vi "Sam_OpenVINO.vi"() -> ()   [LabVIEW 2018]
doc: "Sam_OpenVINO: This example is an example of using the SAM model to achieve semantic segmentation. The SAM model is a semantic segmentation model based on Convolutional Neural Networks (CNN). It adopts technologies such as multi-scale feature fusion and context information encoding, which can achieve pixel level fine segmentation. In this example, by loading the image and clicking on the segmentation area, the segmentation of the region of interest can be achieved."
uses:
  vi.lib/VIRobotics/opencv_yiku/ctls/ColorConversionCodes.ctl
  vi.lib/VIRobotics/opencv_yiku/Mat/Mat_8U/Mat_8U.lvclass
  C:/Program Files/National Instruments/LabVIEW 2018/vi.lib/VIRobotics/opencv_yiku/Mat/Mat/Mat.lvclass
  vi.lib/VIRobotics/ModelZoo/Segmentation/Segment_Anything_OpenVINO/Segment_Anything_OpenVINO.lvclass
  C:/Program Files/National Instruments/LabVIEW 2018/vi.lib/VIRobotics/ModelZoo/Segmentation/Segment_Anything_Utils/Segment_Anything_Utils.lvclass
  vi.lib/VIRobotics/ModelZoo/Segmentation/Segment_Anything_OpenVINO/InitialModel_Segment_Anything_OpenVINO.vi
  vi.lib/VIRobotics/opencv_yiku/Mat/Create_Mat_8U.vi
  vi.lib/VIRobotics/ModelZoo/Segmentation/Segment_Anything_Utils/set_point_coords.vi
  vi.lib/VIRobotics/opencv_yiku/Mat/Create_Mat_8UC3_Size.vi
  vi.lib/VIRobotics/opencv_yiku/Mat/Mat/Mat_release.vi
  vi.lib/VIRobotics/opencv_yiku/Mat/Mat/Mat.lvclass
  vi.lib/VIRobotics/opencv_yiku/opencv_yiku.lvlib
  vi.lib/VIRobotics/ModelZoo/Segmentation/Segment_Anything_Utils/Segment_Anything_Utils.lvclass
panel:
  in  "decodr_config":cluster{"decoder_model":path, "device":string}={"decoder_model"=path "C:/ProgramData/VIRobotics/ModelZoo/Segmentation/sam/sam-b-dec.onnx", "device"="CPU"}
  in  "encoder_config":cluster{"encoder_model":path, "device":string}={"encoder_model"=path "C:/ProgramData/VIRobotics/ModelZoo/Segmentation/sam/sam-b-enc.onnx", "device"="CPU"}
  in  "img":path=path "C:/ProgramData/VIRobotics/ModelZoo/Segmentation/imgs/plant.jpg"
  out "picture":picture
  out "x-y":dbl
  out "mask":picture
  in  "run":bool
  # "Overview: Demonstrates how to use OpenVINO to load the ONNX model of sam for Semantic segmentation annotation\nRequirements: Windows.\nInstructions: \n1.Run the VI.\n2.Specify the img that requires segmentation annotation。\n3.Click on the target with the mouse on the picture control\n4.Click run"
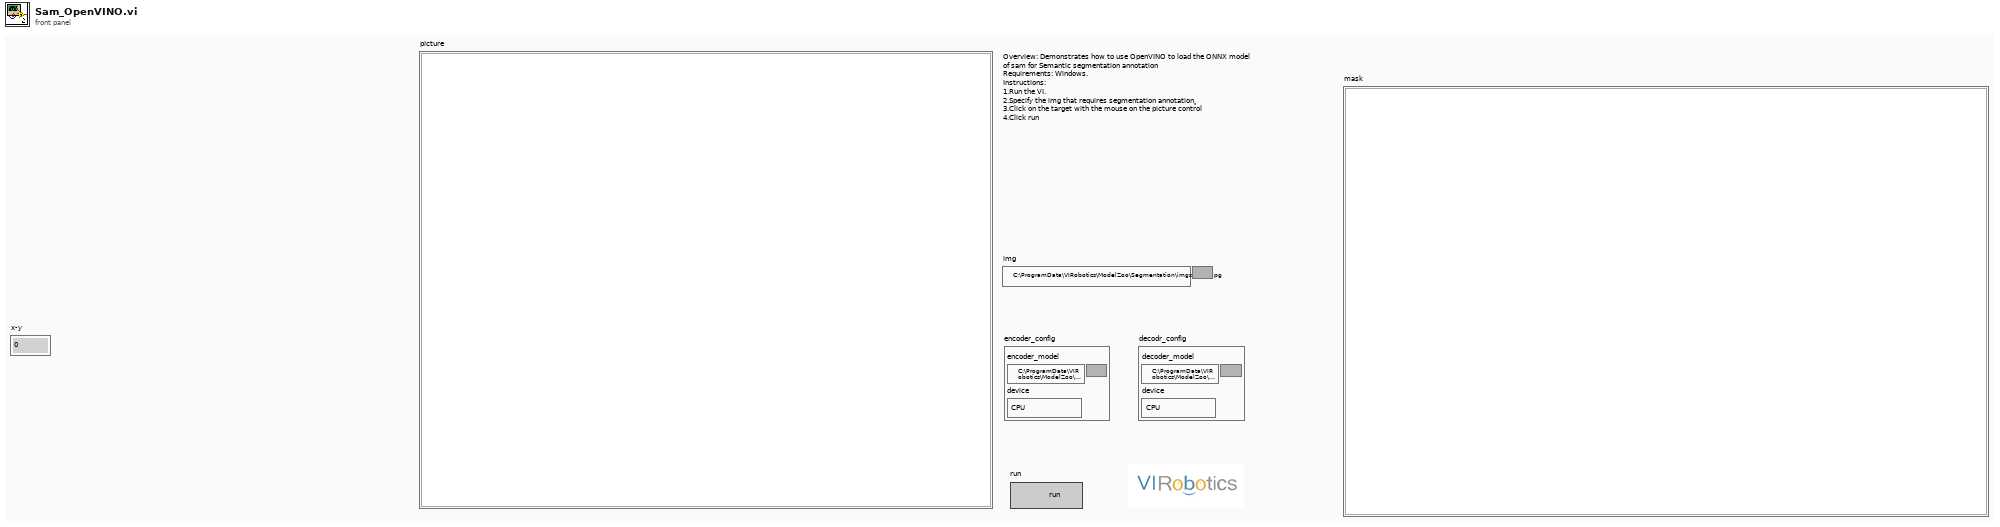
[diagram p1: front panel]
types:
  T1 = typedef "opencv_yiku.lvlib/ColorConversionCodes.ctl" = enum32{"COLOR_BGR2BGRA", "COLOR_BGRA2BGR", "COLOR_BGR2RGBA", "COLOR_RGBA2BGR", "COLOR_BGR2RGB", "COLOR_BGRA2RGBA", "COLOR_BGR2GRAY", "COLOR_RGB2GRAY", "COLOR_GRAY2BGR", "COLOR_GRAY2BGRA", "COLOR_BGRA2GRAY", "COLOR_RGBA2GRAY", "COLOR_BGR2BGR565", "COLOR_RGB2BGR565", "COLOR_BGR5652BGR", "COLOR_BGR5652RGB", "COLOR_BGRA2BGR565", "COLOR_RGBA2BGR565", "COLOR_BGR5652BGRA", "COLOR_BGR5652RGBA", "COLOR_GRAY2BGR565", "COLOR_BGR5652GRAY", "COLOR_BGR2BGR555", "COLOR_RGB2BGR555", "COLOR_BGR5552BGR", "COLOR_BGR5552RGB", "COLOR_BGRA2BGR555", "COLOR_RGBA2BGR555", "COLOR_BGR5552BGRA", "COLOR_BGR5552RGBA", "COLOR_GRAY2BGR555", "COLOR_BGR5552GRAY", "COLOR_BGR2XYZ", "COLOR_RGB2XYZ", "COLOR_XYZ2BGR", "COLOR_XYZ2RGB", "COLOR_BGR2YCrCb", "COLOR_RGB2YCrCb", "COLOR_YCrCb2BGR", "COLOR_YCrCb2RGB", "COLOR_BGR2HSV", "COLOR_RGB2HSV", "42", "43", "COLOR_BGR2Lab", "COLOR_RGB2Lab"}
  T2 = typedef "LVBoundsTypeDef.ctl" = cluster{"Width":u32, "Height":u32}
  T3 = typedef "LVMouseTypeDef.ctl" = cluster{"Mouse Position":cluster{"X":i32, "Y":i32}, "Mouse Modifiers":cluster{"Button Down":bool, "Shift Mod":bool, "Menu Mod":bool, "Option Mod":bool}}
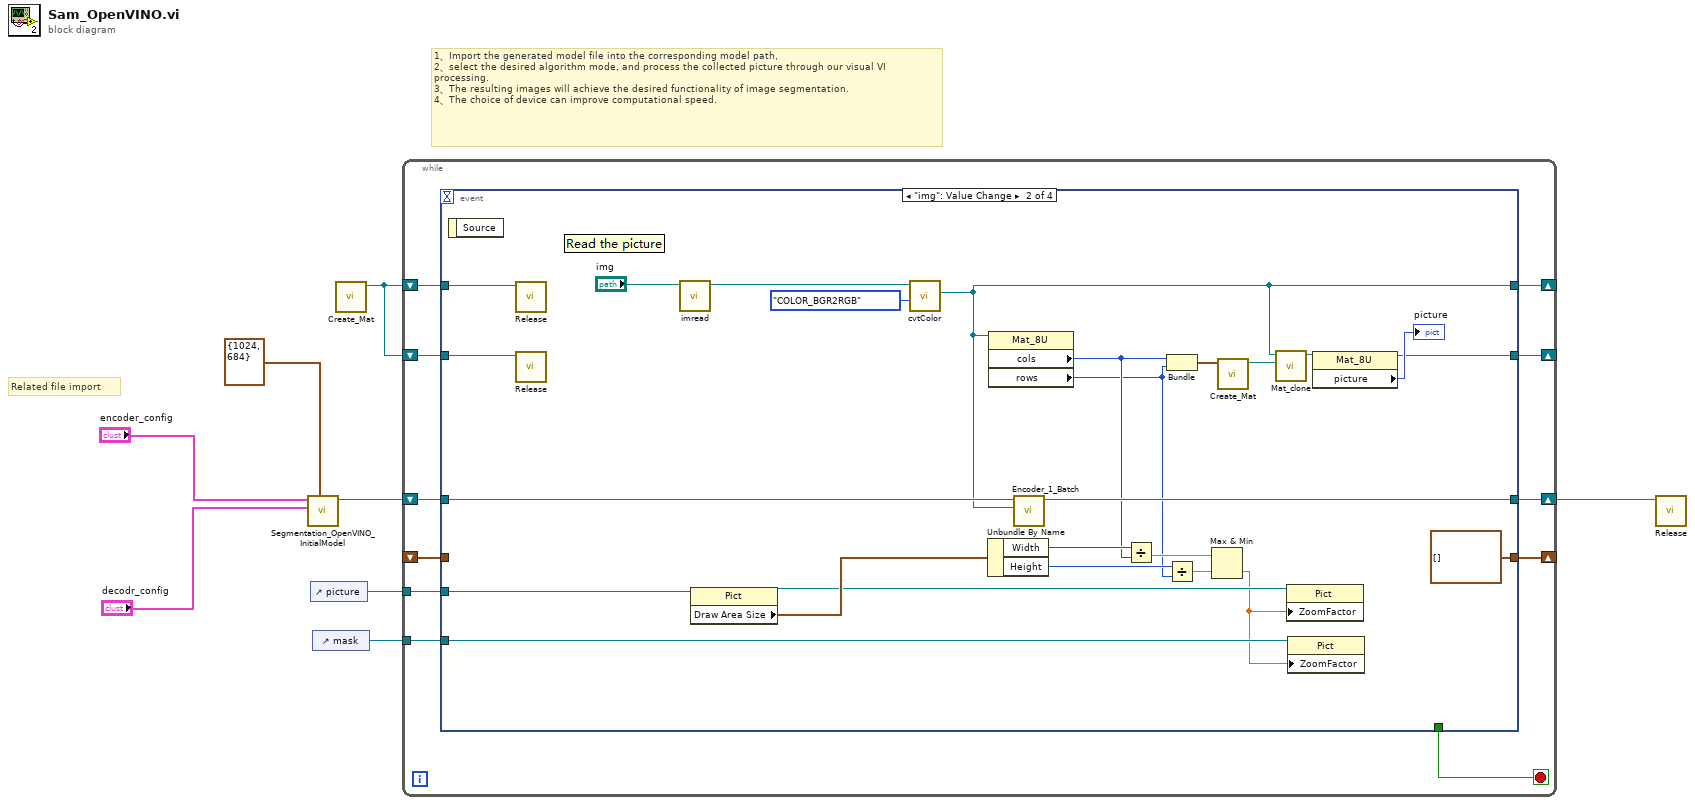
[diagram p0: block diagram]
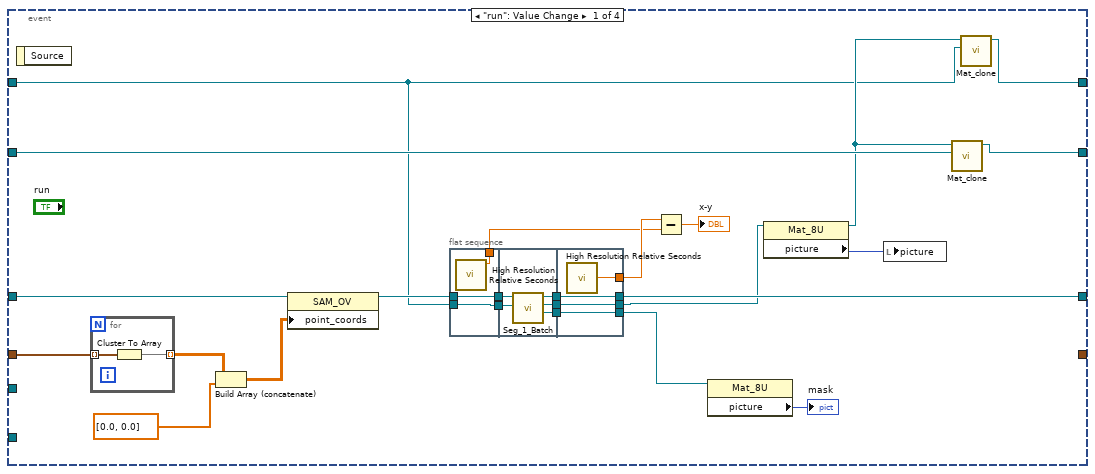
[diagram p2: hidden frame]
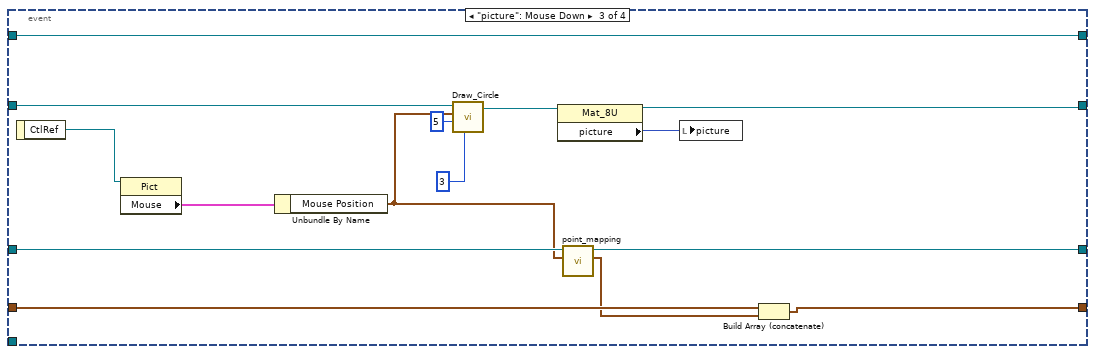
[diagram p3: hidden frame]
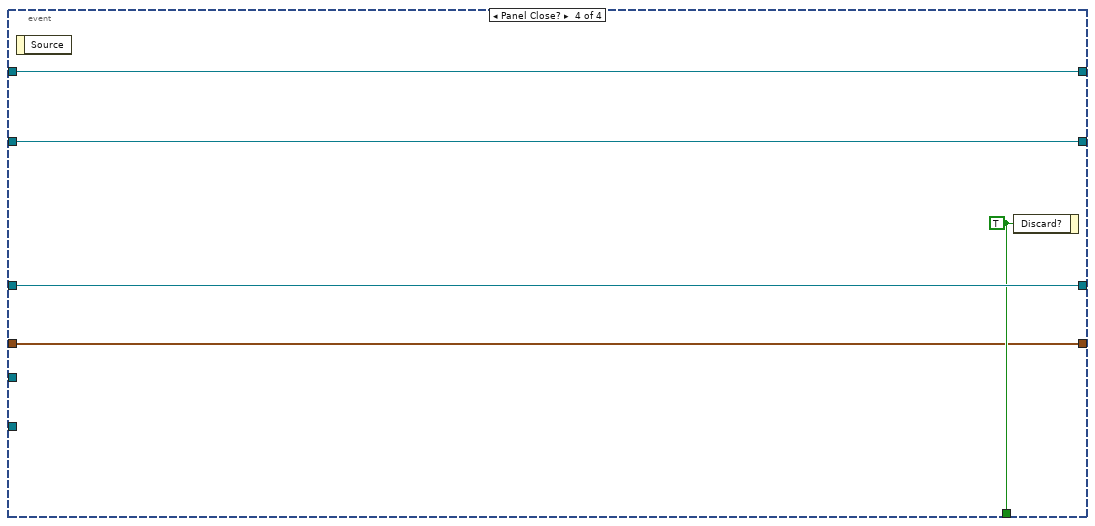
[diagram p4: hidden frame]
diagram:
  # "1、Import the generated model file into the corresponding model path, \n2、select the desired algorithm mode, and process the collected picture through our visual VI processing. \n3、The resulting images will achieve the desired functionality of image segmentation. \n4、The choice of device can improve computational speed."
  # "Related file import"
  n1 = call-poly "Segmentation_OpenVINO_InitialModel.vi"("inputSize"=cluster{"x":i32, "y":i32} {"x"=1024, "y"=684} ("Size"), "decodr_config"="decodr_config", "encoder_config"="encoder_config") -> ("SAM_OV out"=w4:refnum<class "Segment_Anything_OpenVINO.lvclass">)  [unwired: 7 in, 1 out]
  n2 = control-ref of="picture"() -> (w7:refnum<vi>)
  n3 = control-ref of="mask"() -> (w6:refnum<vi>)
  n4 = call-poly "Create_Mat.vi"() -> ("Mat_8U_out"=w5:refnum<class "Mat_8U.lvclass">)  [unwired: 10 in, 1 out]
  n5 = while {
    shift-right: [w18] -> w8
    shift-left: w4 -> [w19]
    tunnel: w7 -> [w16]
    shift-right: [w15] -> _
    shift-left: w5 -> [w14]
    tunnel: w6 -> [w13]
    shift-right: [w12] -> _
    shift-left: _ -> [w11]
    shift-right: [w10] -> _
    shift-left: w5 -> [w9]
    stop <- w17 stop-if-true
    n6 = event shown="[1] \"img\": Value Change" {
      selector: _ -> [_ _ _ _]
      dyn-events: _ -> [_ _ _ _]
      timeout: _ -> [_ _ _ _]
      tunnel: w19 -> [w34 w81 w86 w102]
      tunnel: [w32 w80 w85 w102] -> w18
      tunnel: [_ _ _ w101] -> w17
      tunnel: w16 -> [_ w77 _ _]
      tunnel: [w21 w64 w96 w99] -> w15
      tunnel: w14 -> [w22 w70 w96 w99]
      tunnel: w13 -> [_ w59 _ _]
      tunnel: [_ cluster{"x":sgl, "y":sgl}[] [] w89 w100] -> w12
      tunnel: w11 -> [w31 _ w90 w100]
      tunnel: [w24 w61 w87 w98] -> w10
      tunnel: w9 -> [w25 w60 w88 w98]
      event "run": Value Change {
        n7 = event-data() -> ()  [unwired: 1 in, 1 out]
        n8 = for {
          tunnel: w31 -> [w45] mode=indexing
          tunnel: [w44] -> w30 mode=indexing
          n9 = Cluster To Array(cluster=w45) -> (array=w44:sgl[])
        }
        n10 = Build Array (concatenate)(w30, sgl[] [0.0, 0.0] ("array")) -> (w20:sgl[][])
        n11 = property class="SAM_OV"(reference=w34, "point_coords"=w20) -> (reference out=w33:refnum<class "Segment_Anything_OpenVINO.lvclass">)  [unwired: 1 in, 1 out]
        n12 = flat-sequence {
          tunnel: w33 -> [w48]
          tunnel: [w48] -> w43
          tunnel: [w47] -> w38
          tunnel: w22 -> [w46]
          tunnel: [w46] -> w28
          tunnel: w43 -> [w53]
          tunnel: [w52] -> w42
          tunnel: [w51] -> w41
          tunnel: [w50] -> w40
          tunnel: w28 -> [w49]
          tunnel: [w56] -> w27
          tunnel: [w57] -> w32
          tunnel: w42 -> [w57]
          tunnel: w41 -> [w56]
          tunnel: [w55] -> w39
          tunnel: [w54] -> w36
          tunnel: w40 -> [w54]
          frame #0 {
            n13 = call <vilib>:"High Resolution Relative Seconds.vi"() -> ("relative seconds"=w47:dbl)
          }
          frame #1 {
            n14 = call-dynamic "Seg_1_Batch.vi"("img"=w49, "Segment_Anything_OpenVINO in"=w53) -> ("mask"=w50:refnum<class "Mat_8U.lvclass">, "img out"=w51:refnum<class "Mat_8U.lvclass">, "Segment_Anything_OpenVINO out"=w52:refnum<class "Segment_Anything_OpenVINO.lvclass">)  [unwired: 6 in, 1 out]
          }
          frame #2 {
            n15 = call <vilib>:"High Resolution Relative Seconds.vi"() -> ("relative seconds"=w55:dbl)
          }
        }
        n16 = Subtract(x=w39, y=w38) -> (x-y=→"x-y":dbl)
        n17 = property class="Mat_8U"(reference=w36) -> ("picture"=→"mask":picture)  [unwired: 1 in, 2 out]
        n18 = property class="Mat_8U"(reference=w27) -> (reference out=w23:refnum<class "Mat_8U.lvclass">, "picture"=w26:picture)  [unwired: 1 in, 1 out]
        n19 = local write "picture"(w26) -> ()
        n20 = call "Mat_clone.vi"("dst"=w25, "Mat in"=w23) -> ("dst 2"=w24:refnum<class "Mat_8U.lvclass">)  [unwired: 8 in, 1 out]
        n21 = call "Mat_clone.vi"("dst"=w22, "Mat in"=w23) -> ("dst 2"=w21:refnum<class "Mat_8U.lvclass">)  [unwired: 8 in, 1 out]
      }
      event "img": Value Change {
        n22 = event-data() -> ()  [unwired: 1 in, 1 out]
        n23 = call-poly "Release.vi"("Mat in"=w70) -> ()  [unwired: 10 in, 1 out]
        n24 = call-poly "Release.vi"("Mat in"=w60) -> ()  [unwired: 10 in, 1 out]
        n25 = call "imread.vi"("path"="img") -> ("Mat out"=w79:refnum<class "Mat_8U.lvclass">)  [unwired: 9 in, 1 out]
        n26 = property class="Pict"(reference=w77) -> (reference out=w71:refnum<vi>, "Draw Area Size"=w76:T2)  [unwired: 1 in, 1 out]
        n27 = call "cvtColor.vi"("dstCn"=ColorConversionCodes."COLOR_BGR2RGB", "src"=w79) -> ("dst out"=w64:refnum<class "Mat_8U.lvclass">)  [unwired: 7 in, 2 out]
        n28 = Unbundle By Name(w76) -> ("Width"=w75:u32, "Height"=w74:u32)
        n29 = property class="Mat_8U"(reference=w64) -> ("cols"=w68:i32, "rows"=w67:i32)  [unwired: 1 in, 2 out]
        n30 = call-dynamic "Encoder_1_Batch.vi"("image"=w64, "SAM_OV in"=w81) -> ("SAM_OV out"=w80:refnum<class "Segment_Anything_OpenVINO.lvclass">)  [unwired: 8 in, 1 out]
        n31 = Divide(x=w75, y=w68) -> (x/y=w72:dbl)
        n32 = Bundle("cols"=w68, "rows"=w67) -> (w66:cluster{"cols":i32, "rows":i32})  [unwired: 1 in]
        n33 = Divide(x=w74, y=w67) -> (x/y=w73:dbl)
        n34 = Max & Min(x=w72, y=w73) -> (min(x,y)=w58:dbl)  [unwired: 1 out]
        n35 = call-poly "Create_Mat.vi"("Size"=w66) -> ("Mat_8U_out"=w65:refnum<class "Mat_8U.lvclass">)  [unwired: 9 in, 1 out]
        n36 = call "Mat_clone.vi"("dst"=w65, "Mat in"=w64) -> ("dst 2"=w63:refnum<class "Mat_8U.lvclass">)  [unwired: 8 in, 1 out]
        n37 = property class="Pict"(reference=w71, "ZoomFactor"=w58) -> ()  [unwired: 1 in, 2 out]
        n38 = property class="Pict"(reference=w59, "ZoomFactor"=w58) -> ()  [unwired: 1 in, 2 out]
        n39 = property class="Mat_8U"(reference=w63) -> (reference out=w61:refnum<class "Mat_8U.lvclass">, "picture"=→"picture":picture)  [unwired: 1 in, 1 out]
      }
      event "picture": Mouse Down {
        n40 = event-data() -> ("CtlRef"=w97:refnum<vi>)  [unwired: 1 in]
        n41 = property class="Pict"(reference=w97) -> ("Mouse"=w95:T3)  [unwired: 1 in, 2 out]
        n42 = Unbundle By Name(w95) -> ("Mouse Position"=w84:cluster{"X":i32, "Y":i32})
        n43 = call "Draw_Circle.vi"("thickness"=3, "radius"=5, "center"=w84, "Mat"=w88) -> ("Mat out"=w92:refnum<class "Mat_8U.lvclass">)  [unwired: 6 in, 1 out]
        n44 = property class="Mat_8U"(reference=w92) -> (reference out=w87:refnum<class "Mat_8U.lvclass">, "picture"=w91:picture)  [unwired: 1 in, 1 out]
        n45 = call "point_mapping.vi"("picture_point"=w84, "SAM in"=w86) -> ("tensor_point"=w83:cluster{"x":sgl, "y":sgl}, "SAM out"=w85:refnum<class "Segment_Anything_OpenVINO.lvclass">)  [unwired: 7 in, 1 out]
        n46 = local write "picture"(w91) -> ()
        n47 = Build Array (concatenate)(w90, w83) -> (w89:cluster{"x":sgl, "y":sgl}[])
      }
      event Panel Close? {
        w101 = TRUE ("Discard?")
        n48 = event-data() -> ()  [unwired: 1 in, 1 out]
        n49 = event-data("Discard?"=w101) -> ()  [unwired: 1 in, 1 out]
      }
    }
  }
  n50 = call-dynamic "Release.vi"("Segment_Anything_OpenVINO in"=w8) -> ()  [unwired: 9 in, 2 out]
